vi "Serial_communication_simple.vi"(11 "Command":string) -> (3 "flow":sgl format="%.3g")   [LabVIEW 2015]
uses:
  Program Files (x86)/National Instruments/LabVIEW 2015/examples/Instrument IO/Serial/support/Serial - Settings.ctl
  SubVI/MFC_Address.ctl
  <vilib>/Instr/_visa.llb/VISA Configure Serial Port (Instr).vi
panel:
  out "Response":T1
  out "bytes read":u32
  in  "Serial Settings":T2={"baud rate"=9600, "data bits"=8, "parity"=enum."None", "stop bits"=10, "flow control"=0} {"flow control" items=["None"=0, "XON/XOFF"=1, "RTS/CTS"=2, "DTR/DSR"=4]; "stop bits" items=["1.0"=10, "1.5"=15, "2.0"=20]; "data bits" min=5 max=8 step=1; "baud rate" items=["75"=75, "110"=110, "134"=134, "150"=150, "300"=300, "600"=600, "1200"=1200, "1800"=1800, "2400"=2400, "4800"=4800, "7200"=7200, "9600"=9600, "14400"=14400, "19200"=19200, "28800"=28800, "38400"=38400, "56000"=56000, "57600"=57600, "115200"=115200, "128000"=128000, "230400"=230400]}
  in  "종료문자활성화":bool=TRUE caption="종료 문자\n활성화(참)"
  in  "Port":refnum<visa-resource-name>="COM1"
  out "Error Out":errorcluster caption="에러 출력"
  in  "Error In":errorcluster caption="에러 입력"
  in  "delay (ms)":u32=500
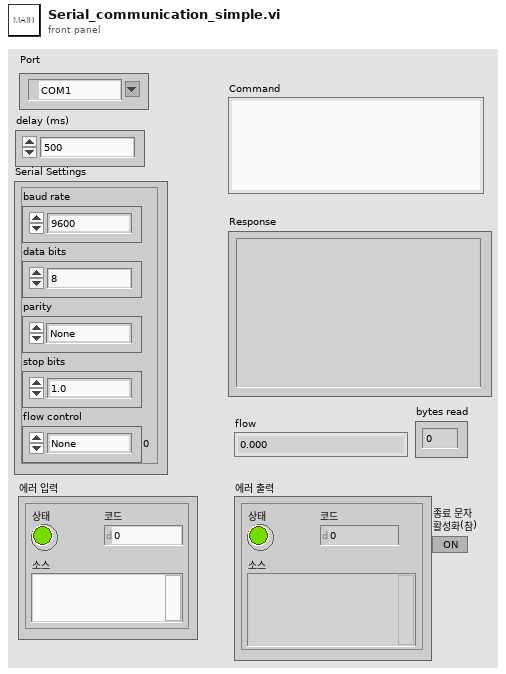
[diagram p1: front panel]
types:
  T1 = typedef "MFC_Address.ctl" = string
  T2 = typedef "Serial - Settings.ctl" = cluster{"baud rate":u32, "data bits":u16, "parity":enum16{"None", "Odd", "Even", "Mark", "Space"}, "stop bits":u16, "flow control":u16}
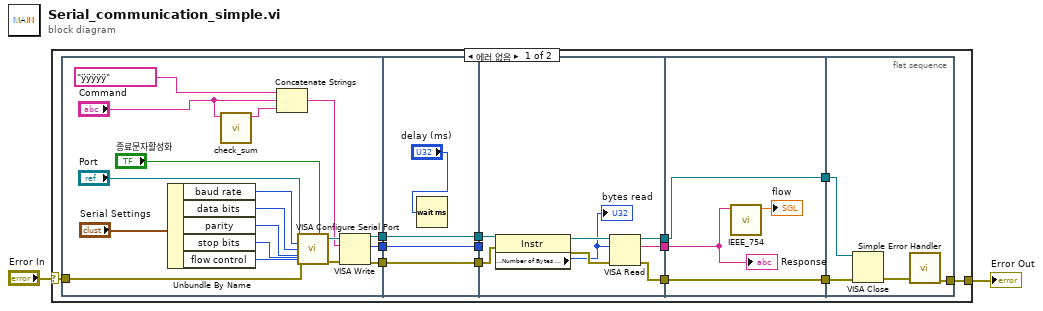
[diagram p0: block diagram]
diagram:
  n1 = case shown="에러 없음" "Error In" {
    selector: "Error In" -> [w3 w54]
    tunnel: [w4 w54] -> w1
    frame No Error {
      n2 = flat-sequence {
        tunnel: [w21] -> w15
        tunnel: [w20] -> w14
        tunnel: [w19] -> w13
        tunnel: w3 -> [w18]
        tunnel: w15 -> [w35]
        tunnel: w14 -> [w37]
        tunnel: w13 -> [w36]
        tunnel: [w37] -> w12
        tunnel: [w36] -> w11
        tunnel: [w35] -> w10
        tunnel: w12 -> [w42]
        tunnel: w11 -> [_]
        tunnel: w10 -> [w41]
        tunnel: [w40] -> w9
        tunnel: [w39] -> w7
        tunnel: [w38] -> w5
        tunnel: w9 -> [w49]
        tunnel: [w49] -> w8
        tunnel: w7 -> [w47]
        tunnel: [w48] -> w6
        tunnel: w5 -> [w48]
        tunnel: w8 -> [w51]
        tunnel: w6 -> [w52]
        tunnel: [w50] -> w4
        frame #0 {
          n3 = Unbundle By Name("Serial Settings") -> ("baud rate"=w27:u32, "data bits"=w26:u16, "parity"=w25:enum16{"None", "Odd", "Even", "Mark", "Space"}, "stop bits"=w24:u16, "flow control"=w23:u16)
          n4 = call "check_sum.vi"("command"="Command") -> ("Check Sum"=w16:string)  [unwired: 10 in]
          n5 = Concatenate Strings("ÿÿÿÿÿ" ("문자열"), "Command", w16) -> (w29:string)
          n6 = call-poly "VISA Configure Serial Port"("VISA resource name"="Port", "Enable Termination\nChar (T)"="종료문자활성화", "baud rate (9600)"=w27, "data bits (8)"=w26, "parity (0:none)"=w25, "error in (no error)"=w18, "stop bits (10: 1 bit)"=w24, "flow control (0:none)"=w23) -> ("VISA resource name out"=w31:refnum<visa-resource-name>, "error out"=w32:errorcluster)  [unwired: 1 in, 5 out]
          n7 = VISA Write(VISA resource name=w31, write buffer=w29, error in (no error)=w32) -> (VISA resource name out=w21:refnum<visa-resource-name>, return count=w19:u32, error out=w20:errorcluster)
        }
        frame #1 {
          n8 = Wait (ms)(milliseconds to wait="delay (ms)") -> ()  [unwired: 1 out]
        }
        frame #2 {
          n9 = property class="Instr"(reference=w41, error in=w42) -> (reference out=w45:refnum<visa-resource-name>, error out=w44:errorcluster, "Serial Settings:Number of Bytes at Serial Port"=w43:u32)
          "bytes read" <- w43
          n10 = VISA Read(VISA resource name=w45, byte count=w43, error in (no error)=w44) -> (VISA resource name out=w38:refnum<visa-resource-name>, read buffer=w39:string, error out=w40:errorcluster)  [unwired: 1 out]
        }
        frame #3 {
          n11 = call "IEEE_754.vi"("input"=w47) -> ("Return"=→"flow":sgl)  [unwired: 10 in]
          "Response" <- w47
        }
        frame #4 {
          n12 = VISA Close(VISA resource name=w52, error in (no error)=w51) -> (error out=w53:errorcluster)
          n13 = call <vilib>:"Simple Error Handler.vi"("error in (no error)"=w53) -> ("error out"=w50:errorcluster)  [unwired: 1 in, 7 out]
        }
      }
    }
    frame Error {
    }
  }
  "Error Out" <- w1
